vi "Acquire.vi"(8 "error in (no error)":errorcluster, 11 "Frequency Measurement in":refnum<class "Frequency Measurement.lvclass">) -> (0 "error out":errorcluster, 3 "Frequency Measurement out":refnum<class "Frequency Measurement.lvclass">)   [LabVIEW 2015, in "Frequency Measurement.lvlib" / "Frequency Measurement.lvclass"]
uses:
  Frequency Measurement.lvclass
  <userlib>/Common Components/Hardware/Scope/Scope.lvclass
  <userlib>/Common Components/Hardware/FGEN/Function Generator.lvclass
  <vilib>/ActorFramework/Actor/Actor.lvclass/Actor.ctl
  <vilib>/ActorFramework/Message Enqueuer/Message Enqueuer.lvclass/Message Enqueuer.ctl
  <vilib>/ActorFramework/Message Enqueuer/Init from Existing Queue.vi
  <vilib>/ActorFramework/Message Enqueuer/Enqueue.vi
  <vilib>/ActorFramework/Message Priority Queue/Priority Enqueue.vi
  <vilib>/ActorFramework/Message Enqueuer/Message Enqueuer.lvclass
  <userlib>/Common Components/Measurement Actor/Messages/Measure Msg/Measure Msg.lvclass
  <userlib>/Common Components/Measurement Actor/Measurement.lvclass
  <vilib>/ActorFramework/Actor/Actor.lvclass
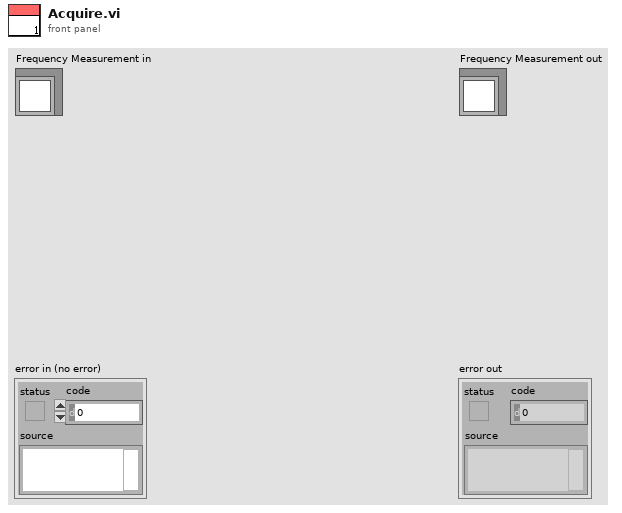
[diagram p1: front panel]
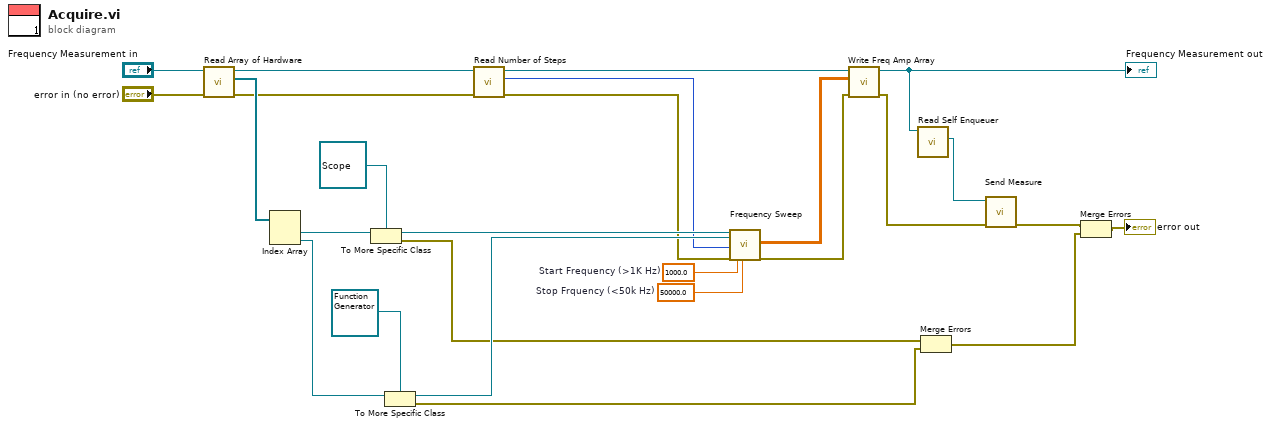
[diagram p0: block diagram]
diagram:
  w20 = 1000.0  # Start Frequency (>1K Hz)
  w21 = 50000.0  # Stop Frquency (<50k Hz)
  n1 = call <userlib>:"Read Array of Hardware.vi"("error in (no error)"="error in (no error)", "Measurement in"="Frequency Measurement in") -> ("error out"=w10:errorcluster, "Array of Hardware"=w24:refnum<class "Hardware.lvclass">[], "Measurement out"=w17:refnum<class "Frequency Measurement.lvclass">)  [unwired: 7 in]
  n2 = Index Array(array=w24) -> (element #1=w26:refnum<class "Hardware.lvclass">, element #2=w25:refnum<class "Hardware.lvclass">)  [unwired: 2 in]
  n3 = To More Specific Class(target class=refnum<class "Scope.lvclass"> refnum ("Hardware.lvlib:Scope.lvclass"), reference=w26) -> (specific class reference=w23:refnum<class "Scope.lvclass">, error out=w9:errorcluster)  [unwired: 1 in]
  n4 = To More Specific Class(target class=refnum<class "Function Generator.lvclass"> refnum ("Hardware.lvlib:Function Generator.lvclass"), reference=w25) -> (specific class reference=w22:refnum<class "Function Generator.lvclass">, error out=w8:errorcluster)  [unwired: 1 in]
  n5 = call "Read Number of Steps.vi"("error in (no error)"=w10, "Frequency Measurement in"=w17) -> ("error out"=w11:errorcluster, "Number of Steps"=w18:i32, "Frequency Measurement out"=w16:refnum<class "Frequency Measurement.lvclass">)  [unwired: 7 in]
  n6 = call "Frequency Sweep.vi"("Hardware.lvlib:Scope.lvclass"=w23, "Hardware.lvlib:Function Generator.lvclass"=w22, "Number of Steps (25)"=w18, "error in (no error)"=w11, "Start Frequency (1000)"=w20, "Stop Frequency (50000)"=w21) -> ("Freq Amp Array"=w19:dbl[][], "error out"=w12:errorcluster)  [unwired: 10 in, 2 out]
  n7 = call "Write Freq Amp Array.vi"("error in (no error)"=w12, "Freq Amp Array"=w19, "Frequency Measurement in"=w16) -> ("error out"=w13:errorcluster, "Frequency Measurement out"=w4:refnum<class "Frequency Measurement.lvclass">)  [unwired: 7 in]
  "Frequency Measurement out" <- w4
  n8 = call <vilib>:"Read Self Enqueuer.vi"("Actor"=w4) -> ("Self Enqueuer"=w3:refnum<class "Message Enqueuer.lvclass">)  [unwired: 10 in]
  n9 = Merge Errors(w9, w8) -> (w6:errorcluster)
  n10 = call <userlib>:"Send Measure.vi"("error in (no error)"=w13, "Message Enqueuer in"=w3) -> ("error out"=w7:errorcluster)  [unwired: 8 in, 1 out]
  n11 = Merge Errors(w7, w6) -> (→"error out":errorcluster)
